vi "Table Interpolation.vi"(7 "Invert":bool, 8 "Z":dbl, 9 "Y":dbl, 10 "X":dbl, 11 "Table":T1) -> (0 "a":dbl, 1 "z":dbl, 2 "y":dbl, 3 "x":dbl)   [LabVIEW 2013]
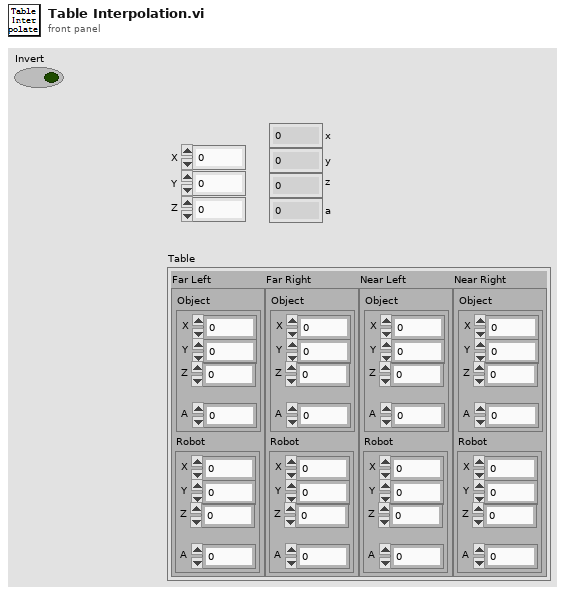
[diagram p1: front panel]
types:
  T1 = cluster{"Far Left":cluster{"Object":cluster{"X":dbl, "Y":dbl, "Z":dbl, "A":dbl}, "Robot":cluster{"X":dbl, "Y":dbl, "Z":dbl, "A":dbl}}, "Far Right":cluster{"Object":cluster{"X":dbl, "Y":dbl, "Z":dbl, "A":dbl}, "Robot":cluster{"X":dbl, "Y":dbl, "Z":dbl, "A":dbl}}, "Near Left":cluster{"Object":cluster{"X":dbl, "Y":dbl, "Z":dbl, "A":dbl}, "Robot":cluster{"X":dbl, "Y":dbl, "Z":dbl, "A":dbl}}, "Near Right":cluster{"Object":cluster{"X":dbl, "Y":dbl, "Z":dbl, "A":dbl}, "Robot":cluster{"X":dbl, "Y":dbl, "Z":dbl, "A":dbl}}}
  T2 = cluster{"Object":cluster{"X":dbl, "Y":dbl, "Z":dbl, "A":dbl}, "Robot":cluster{"X":dbl, "Y":dbl, "Z":dbl, "A":dbl}}
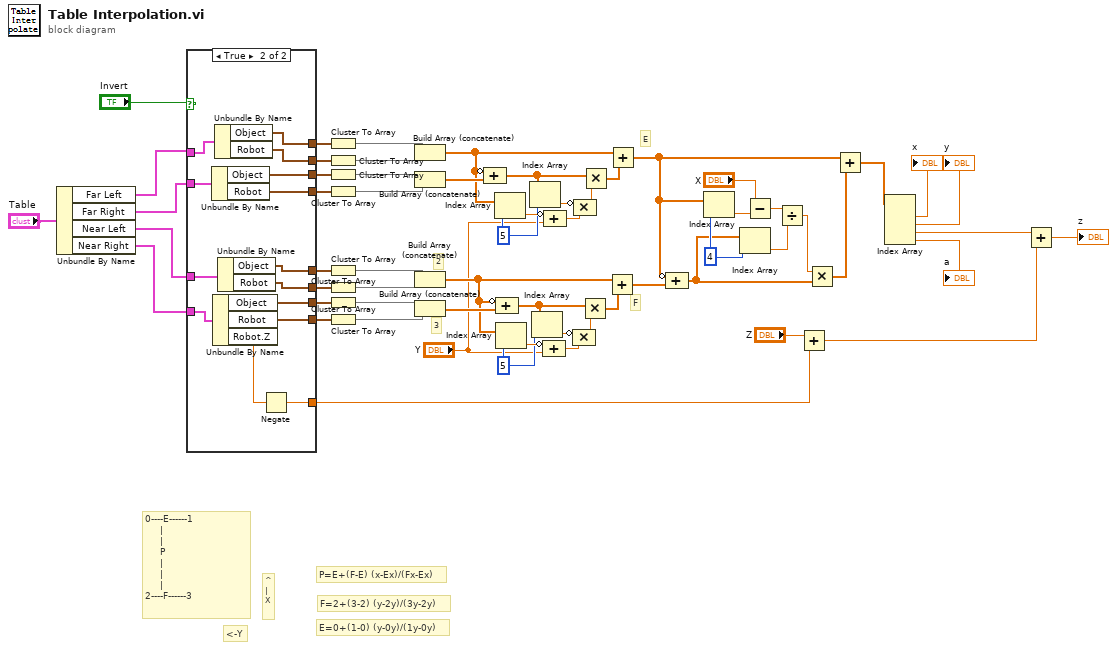
[diagram p0: block diagram]
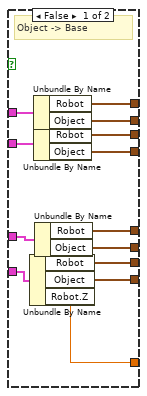
[diagram p2: hidden frame]
diagram:
  w31 = 4 ("index")
  w33 = 5 ("index")
  w34 = 5 ("index")
  # "E=0+(1-0) (y-0y)/(1y-0y)"
  # "3"
  # "2"
  # "F=2+(3-2) (y-2y)/(3y-2y)"
  # "P=E+(F-E) (x-Ex)/(Fx-Ex)"
  # "F"
  # "E"
  # "^\n|\nX"
  # "<-Y"
  # "0----E------1\n     |    \n     |       \n     P\n     |\n     |\n     |\n2----F------3"
  n1 = Unbundle By Name("Table") -> ("Far Left"=w57:T2, "Far Right"=w56:T2, "Near Left"=w55:T2, "Near Right"=w54:T2)
  n2 = case shown="True" "Invert" {
    tunnel: w56 -> [w73 w87]
    tunnel: w54 -> [w72 w86]
    tunnel: [w71 w81] -> w59
    tunnel: [w70 w85] -> w48
    tunnel: [w69 w84] -> w49
    tunnel: [w68 w80] -> w58
    tunnel: [w63 w79] -> w53
    tunnel: [w67 w83] -> w50
    tunnel: [w66 w82] -> w51
    tunnel: [w62 w78] -> w52
    tunnel: w57 -> [w65 w76]
    tunnel: w55 -> [w64 w77]
    tunnel: [w61 w74] -> w3
    frame False {
      # "Object -> Base"
      n3 = Unbundle By Name(w72) -> ("Robot"=w66:cluster{"X":dbl, "Y":dbl, "Z":dbl, "A":dbl}, "Object"=w67:cluster{"X":dbl, "Y":dbl, "Z":dbl, "A":dbl}, "Robot.Z"=w61:dbl)
      n4 = Unbundle By Name(w65) -> ("Robot"=w71:cluster{"X":dbl, "Y":dbl, "Z":dbl, "A":dbl}, "Object"=w68:cluster{"X":dbl, "Y":dbl, "Z":dbl, "A":dbl})
      n5 = Unbundle By Name(w73) -> ("Robot"=w69:cluster{"X":dbl, "Y":dbl, "Z":dbl, "A":dbl}, "Object"=w70:cluster{"X":dbl, "Y":dbl, "Z":dbl, "A":dbl})
      n6 = Unbundle By Name(w64) -> ("Robot"=w63:cluster{"X":dbl, "Y":dbl, "Z":dbl, "A":dbl}, "Object"=w62:cluster{"X":dbl, "Y":dbl, "Z":dbl, "A":dbl})
    }
    frame True {
      n7 = Unbundle By Name(w87) -> ("Object"=w84:cluster{"X":dbl, "Y":dbl, "Z":dbl, "A":dbl}, "Robot"=w85:cluster{"X":dbl, "Y":dbl, "Z":dbl, "A":dbl})
      n8 = Unbundle By Name(w86) -> ("Object"=w82:cluster{"X":dbl, "Y":dbl, "Z":dbl, "A":dbl}, "Robot"=w83:cluster{"X":dbl, "Y":dbl, "Z":dbl, "A":dbl}, "Robot.Z"=w75:dbl)
      n9 = Unbundle By Name(w76) -> ("Object"=w81:cluster{"X":dbl, "Y":dbl, "Z":dbl, "A":dbl}, "Robot"=w80:cluster{"X":dbl, "Y":dbl, "Z":dbl, "A":dbl})
      n10 = Unbundle By Name(w77) -> ("Object"=w79:cluster{"X":dbl, "Y":dbl, "Z":dbl, "A":dbl}, "Robot"=w78:cluster{"X":dbl, "Y":dbl, "Z":dbl, "A":dbl})
      n11 = Negate(x=w75) -> (-x=w74:dbl)
    }
  }
  n12 = Cluster To Array(cluster=w59) -> (array=w24:dbl[])
  n13 = Cluster To Array(cluster=w58) -> (array=w23:dbl[])
  n14 = Cluster To Array(cluster=w49) -> (array=w22:dbl[])
  n15 = Cluster To Array(cluster=w48) -> (array=w21:dbl[])
  n16 = Cluster To Array(cluster=w53) -> (array=w20:dbl[])
  n17 = Cluster To Array(cluster=w52) -> (array=w19:dbl[])
  n18 = Cluster To Array(cluster=w51) -> (array=w18:dbl[])
  n19 = Cluster To Array(cluster=w50) -> (array=w17:dbl[])
  n20 = Build Array (concatenate)(w24, w23) -> (w27:dbl[])
  n21 = Build Array (concatenate)(w22, w21) -> (w47:dbl[])
  n22 = Build Array (concatenate)(w20, w19) -> (w28:dbl[])
  n23 = Build Array (concatenate)(w18, w17) -> (w29:dbl[])
  n24 = Compound Arithmetic op=ADD(invert w27, w47) -> (w43:dbl[])
  n25 = Index Array(array=w27, index=w33) -> (element=w46:dbl)
  n26 = Compound Arithmetic op=ADD(invert w28, w29) -> (w37:dbl[])
  n27 = Index Array(array=w28, index=w34) -> (element=w40:dbl)
  n28 = Index Array(array=w43, index=w33) -> (element=w44:dbl)
  n29 = Index Array(array=w37, index=w34) -> (element=w38:dbl)
  n30 = Compound Arithmetic op=ADD(invert w40, "Y") -> (w39:dbl)
  n31 = Compound Arithmetic op=ADD(invert w46, "Y") -> (w45:dbl)
  n32 = Compound Arithmetic op=MULTIPLY(invert w38, w39) -> (w36:dbl)
  n33 = Compound Arithmetic op=MULTIPLY(invert w44, w45) -> (w42:dbl)
  n34 = Multiply(x=w37, y=w36) -> (x*y=w35:dbl[])
  n35 = Multiply(x=w43, y=w42) -> (x*y=w41:dbl[])
  n36 = Add(x=w28, y=w35) -> (x+y=w30:dbl[])
  n37 = Add(x=w27, y=w41) -> (x+y=w26:dbl[])
  n38 = Compound Arithmetic op=ADD(invert w26, w30) -> (w12:dbl[])
  n39 = Index Array(array=w26, index=w31) -> (element=w8:dbl)
  n40 = Index Array(array=w12, index=w31) -> (element=w10:dbl)
  n41 = Subtract(x="X", y=w8) -> (x-y=w9:dbl)
  n42 = Divide(x=w9, y=w10) -> (x/y=w11:dbl)
  n43 = Add(x="Z", y=w3) -> (x+y=w2:dbl)
  n44 = Multiply(x=w11, y=w12) -> (x*y=w32:dbl[])
  n45 = Add(x=w26, y=w32) -> (x+y=w16:dbl[])
  n46 = Index Array(array=w16) -> (element #1=→"x":dbl, element #2=→"y":dbl, element #3=w7:dbl, element #4=→"a":dbl)  [unwired: 4 in]
  n47 = Add(x=w7, y=w2) -> (x+y=→"z":dbl)
